vi "ReadXmlFileOnRio.vi"(8 "Motor Id":string="Drive Right Rear", 9 "Robot Id":string="984", 11 "file path (dialog if empty) 2":path=path "C:/git/ViTestFiles/RobotConfiguration-8.xml") -> (2 "Pdp Channel Id":string, 3 "Can Bus ID":string)   [LabVIEW 2016]
uses:
  <vilib>/xml/Load XML File.vi
  <vilib>/xml/NI_XML.lvlib
  <resource>/objmgr/DOMUserDefRef.rc
panel:
  out "Debug Array 2":string[](array[string])
  out "Numeric 2":i32
  out "Numeric 1":i32
  out "Debug Array 1":string[](array[string])
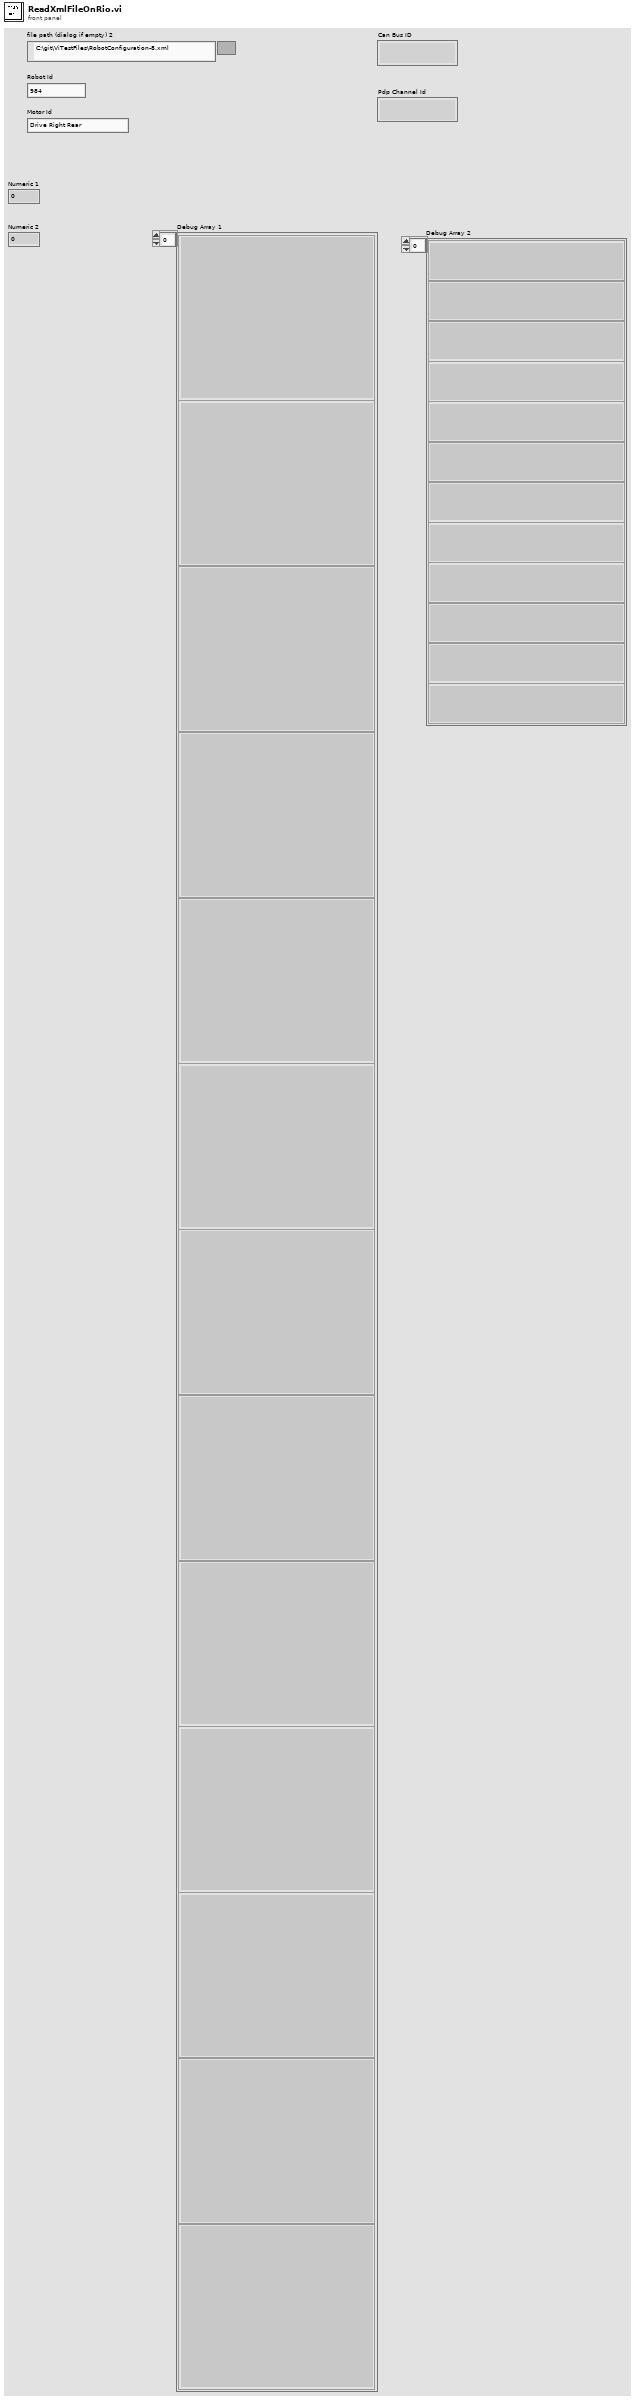
[diagram p1: front panel]
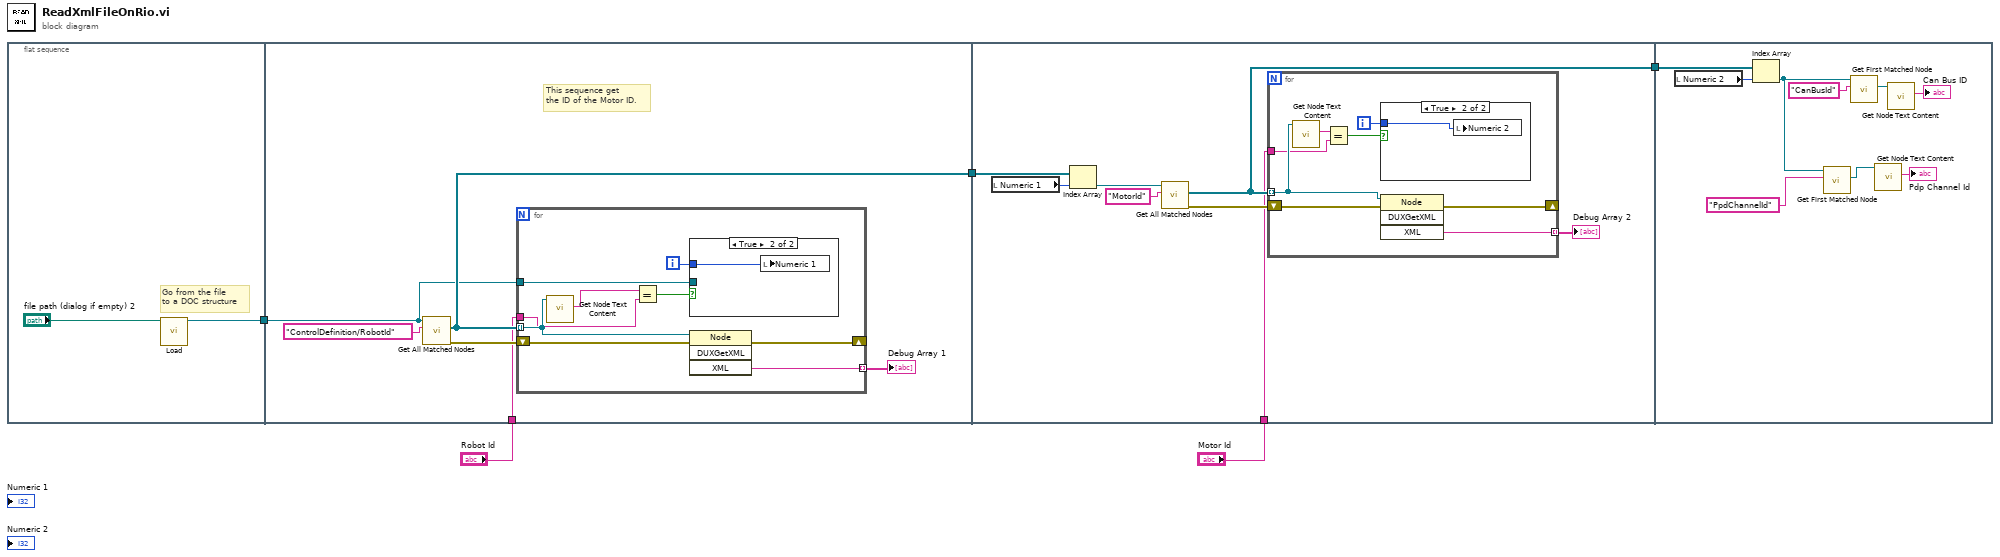
[diagram p0: block diagram]
diagram:
  n1 = flat-sequence {
    tunnel: [w6] -> w5
    tunnel: [w11] -> w4
    tunnel: w5 -> [w9]
    tunnel: "Robot Id" -> [w8]
    tunnel: w4 -> [w29]
    tunnel: [w25] -> w3
    tunnel: "Motor Id" -> [w24]
    tunnel: w3 -> [w49]
    frame #0 {
      # "Go from the file\nto a DOC structure"
      n2 = call-poly <vilib>:"Load.vi"("path to XML document"="file path (dialog if empty) 2") -> ("DOM document out"=w6:refnum<k20>)  [unwired: 12 in, 2 out]
    }
    frame #1 {
      # "This sequence get\nthe ID of the Motor ID."
      n3 = call <vilib>:"Get All Matched Nodes.vi"("XPath expression"="ControlDefinition/RobotId" ("Robot Id xPath"), "node in"=w9) -> ("error out"=w13:errorcluster, "node result array"=w11:refnum<k20>[])  [unwired: 7 in, 1 out]
      n4 = for {
        shift-right: [w20] -> _
        shift-left: w13 -> [w21]
        tunnel: [w22] -> w10 mode=indexing
        tunnel: w11 -> [w19] mode=indexing
        tunnel: w9 -> [w16]
        tunnel: w8 -> [w14]
        i -> [w15]
        n5 = call <vilib>:"Get Node Text Content.vi"("node in"=w19) -> ("node text"=w18:string)  [unwired: 8 in, 2 out]
        n6 = Equal?(x=w18, y=w14) -> (x = y?=w17:bool)
        n7 = case shown="True" w17 {
          tunnel: w16 -> [_ _]
          tunnel: w15 -> [_ w23]
          frame False {
          }
          frame True {
            n8 = local write "Numeric 1"(w23) -> ()
          }
        }
        n9 = invoke on="Invoke Node" class="Node" method="DUXGetXML"(reference=w19, error in=w21) -> (error out=w20:errorcluster, "XML"=w22:string)  [unwired: 2 in, 2 out]
      }
      "Debug Array 1" <- w10
    }
    frame #2 {
      n10 = local read "Numeric 1"() -> (w31:i32)
      n11 = Index Array(array=w29, index=w31) -> (element=w28:refnum<k20>)
      n12 = call <vilib>:"Get All Matched Nodes.vi"("XPath expression"="MotorId" ("Motor Id xPath"), "node in"=w28) -> ("error out"=w27:errorcluster, "node result array"=w25:refnum<k20>[])  [unwired: 7 in, 1 out]
      n13 = for {
        shift-right: [w38] -> _
        shift-left: w27 -> [w39]
        tunnel: w25 -> [w34] mode=indexing
        tunnel: [w33] -> w26 mode=indexing
        tunnel: w24 -> [w32]
        i -> [w35]
        n14 = call <vilib>:"Get Node Text Content.vi"("node in"=w34) -> ("node text"=w37:string)  [unwired: 8 in, 2 out]
        n15 = Equal?(x=w37, y=w32) -> (x = y?=w36:bool)
        n16 = case shown="True" w36 {
          tunnel: w35 -> [_ w40]
          frame False {
          }
          frame True {
            n17 = local write "Numeric 2"(w40) -> ()
          }
        }
        n18 = invoke on="Invoke Node" class="Node" method="DUXGetXML"(reference=w34, error in=w39) -> (error out=w38:errorcluster, "XML"=w33:string)  [unwired: 2 in, 2 out]
      }
      "Debug Array 2" <- w26
    }
    frame #3 {
      n19 = local read "Numeric 2"() -> (w48:i32)
      n20 = Index Array(array=w49, index=w48) -> (element=w43:refnum<k20>)
      n21 = call <vilib>:"Get First Matched Node.vi"("XPath expression"="PpdChannelId", "node in"=w43) -> ("node result"=w44:refnum<k20>)  [unwired: 7 in, 2 out]
      n22 = call <vilib>:"Get First Matched Node.vi"("XPath expression"="CanBusId", "node in"=w43) -> ("node result"=w46:refnum<k20>)  [unwired: 7 in, 2 out]
      n23 = call <vilib>:"Get Node Text Content.vi"("node in"=w44) -> ("node text"=→"Pdp Channel Id":string)  [unwired: 8 in, 2 out]
      n24 = call <vilib>:"Get Node Text Content.vi"("node in"=w46) -> ("node text"=→"Can Bus ID":string)  [unwired: 8 in, 2 out]
    }
  }
